vi "Write Value.vi"(8 "error in (no error)":errorcluster, 10 "Data":T1, 11 "Numeric in":refnum<class "Const_CPLX_DBL.lvclass">) -> (0 "error out":errorcluster, 3 "Numeric out":refnum<class "Const_CPLX_DBL.lvclass">)   [LabVIEW 2021, in "Const_CPLX_DBL.lvclass"]
uses:
  Const_CPLX_DBL.lvclass
  Type.ctl
  Const_CPLX_DBL.lvclass/Const_CPLX_DBL.ctl
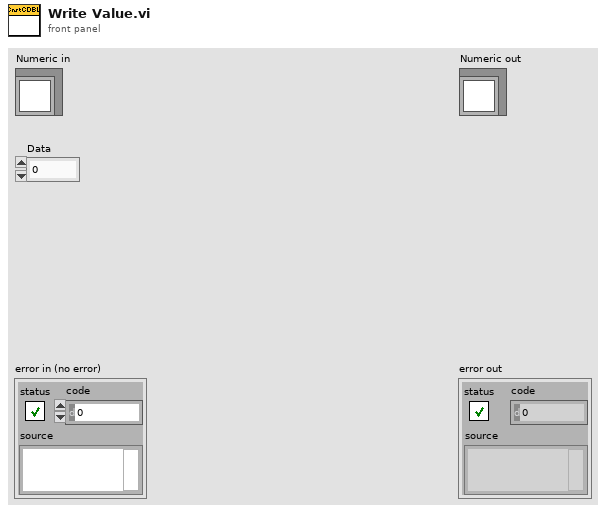
[diagram p1: front panel]
types:
  T1 = typedef "Const_CPLX_DBL.lvclass/Type.ctl" = cdb
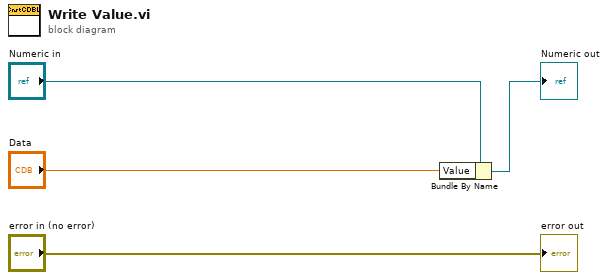
[diagram p0: block diagram]
diagram:
  n1 = Bundle By Name(cluster="Numeric in", "Value"="Data") -> (→"Numeric out":refnum<class "Const_CPLX_DBL.lvclass">)
  "error out" <- "error in (no error)"
